vi "1D Polynomial Evaluation.vi"(2 "Coefficients: a":dbl[](array[numeric]) format="%0.2f", 3 "X":dbl[](array[numeric]) format="%0.2f") -> (0 "error":i32, 1 "Y":dbl[](array[numeric]) format="%0.2f")   [LabVIEW 2010, in "NI_AALBase.lvlib"]
doc: "LabVIEW no longer supports this VI. Use the Polynomial Evaluation VI instead.\nPerforms a polynomial evaluation of <b>X</b> using <b>Coefficients: a</b>.\nThis VI calculates the output array <b>Y</b> using the following equation:\nY = sum(a[n]*X^n, n, 0, m)\nwhere m denotes the polynomial order, n = 0, 1, 2, ..., m, a is the Coefficient array, and m + 1 is the number of coefficients."
uses:
  NI_AALBase.lvlib
  lvanlys.dll
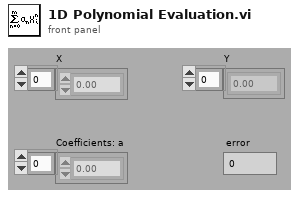
[diagram p1: front panel]
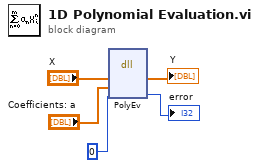
[diagram p0: block diagram]
diagram:
  n1 = dll-call lib="C:/Program Files/National Instruments/LabVIEW 2010/resource/lvanlys.*" fn="PolyEv"("X"="X", "Coefficients: a"="Coefficients: a", 0) -> ("X"=→"Y":dbl[], →"error":i32)  [unwired: 5 in, 2 out]
